vi "BC Verify Component Configuration.vi"(8 "error in (no error)":errorcluster, 11 "Bus Controller in":refnum<class "Bus Controller.lvclass">) -> (0 "error out":errorcluster, 3 "Bus Controller out":refnum<class "Bus Controller.lvclass">)   [LabVIEW 2020, in "Unit Tests.lvlib" / "Bus Controller.lvclass"]
uses:
  Bus Controller.lvclass
  Bus Controller.lvclass/Bus Controller.ctl
  <vilib>/addons/_JKI Toolkits/Caraya/classes/Assert/Assert True.vi
  Dependencies/FPGA Interface/FPGA Interface.lvclass
  <vilib>/addons/_JKI Toolkits/Caraya/classes/Assert/Assert.lvclass
  <vilib>/addons/_JKI Toolkits/Caraya/classes/Test/Test.lvclass
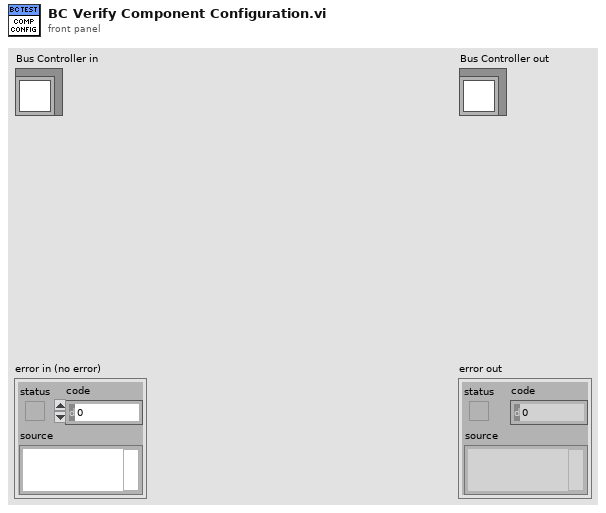
[diagram p1: front panel]
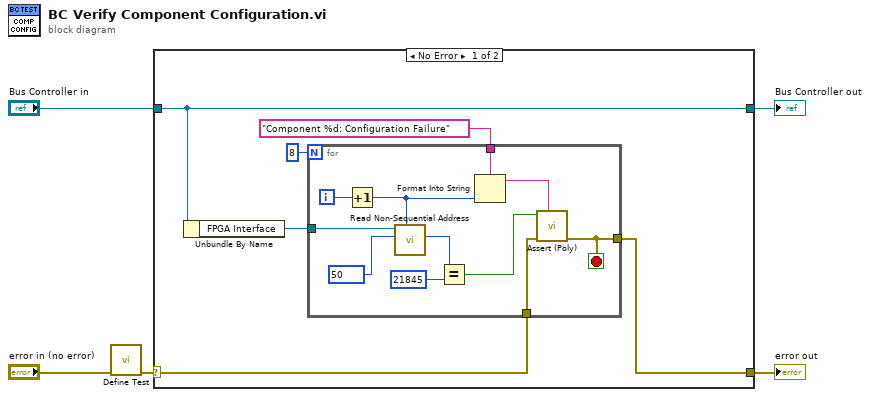
[diagram p0: block diagram]
diagram:
  n1 = call <vilib>:"Define Test.vi"("error in (no error)"="error in (no error)") -> ("error out"=w1:errorcluster)  [unwired: 9 in, 1 out]
  n2 = case shown="No Error" w1 {
    selector: w1 -> [w9 w24]
    tunnel: [w8 w24] -> w5
    tunnel: [w11 w23] -> w3
    tunnel: "Bus Controller in" -> [w11 w23]
    frame No Error {
      n3 = Unbundle By Name(w11) -> ("FPGA Interface"=w10:refnum<class "FPGA Interface.lvclass">)
      n4 = for {
        N: 8 -> [_]
        tunnel: w10 -> [w22]
        tunnel: "Component %d: Configuration Failure" ("custom report message (\"\")") -> [w18]
        tunnel: w9 -> [w13]
        tunnel: [w12] -> w8
        i -> [w21]
        stop <- w12 stop-if-true
        n5 = Increment(x=w21) -> (x+1=w17:i32)
        n6 = call-dynamic "Read Non-Sequential Address.vi"("Target IC (1-8)"=w17, "Address"=u16 50, "FPGA Interface in"=w22) -> ("Data"=w16:u16)  [unwired: 7 in, 1 out]
        n7 = Equal?(x=w16, y=u16 21845) -> (x = y?=w15:bool)
        n8 = Format Into String(format string=w18, w17) -> (resulting string=w14:string)  [unwired: 2 in, 1 out]
        n9 = call-poly <vilib>:"Assert (Poly).vi"("Label"=w14, "error in (no error)"=w13, "True?"=w15) -> ("error out"=w12:errorcluster)  [unwired: 7 in, 1 out]
      }
    }
    frame Error {
    }
  }
  "error out" <- w5
  "Bus Controller out" <- w3
